vi "NTViewerUI.vi"(9 "Client Name":string, 10 "Server IP Address":string="localhost", 11 "StopNotifier":refnum<notifier>) -> ()   [LabVIEW 2015]
panel:
  in  "Tab Control":enum32{"All Table Entries", "User Page 1"}(tab)
  in  "NT Entries":string(tree)
  in  "Robot223/MyDouble2":dbl
  out "MyDouble":dbl
  # "First page of user controls. Here you can add as many controls as you like, as well as create other pages\nfor controls. These will all automatically be bound to the SmartDashboard."
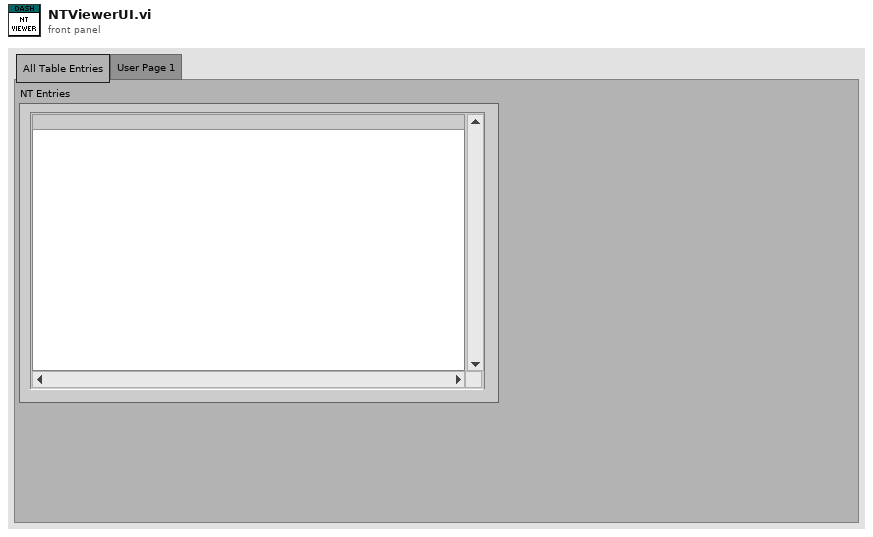
[diagram p1: front panel]
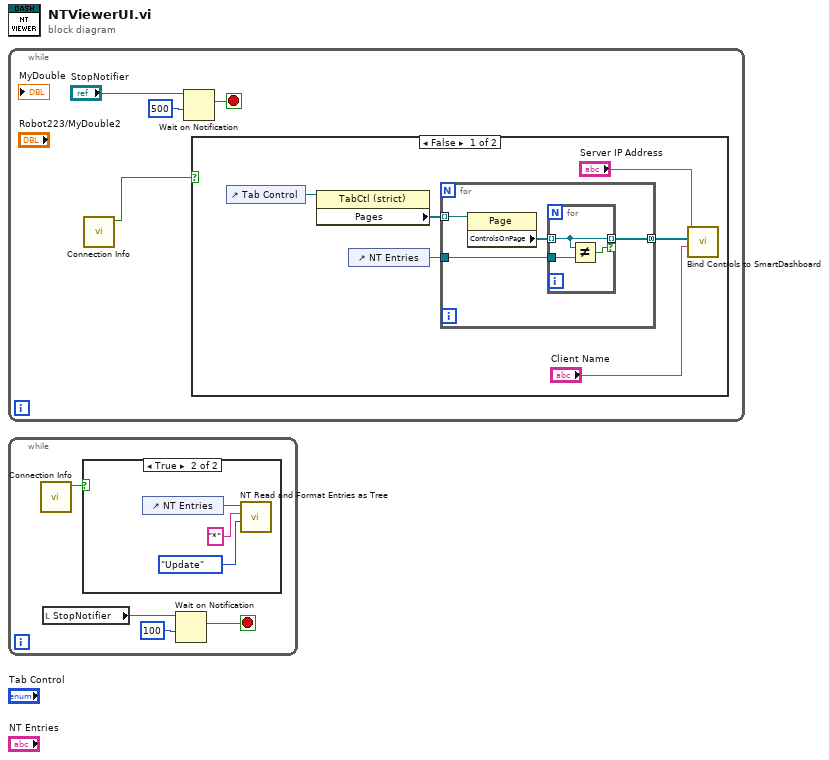
[diagram p0: block diagram]
diagram:
  n1 = while {
    stop <- w2 stop-if-true
    n2 = call <vilib>:"Connection Info.vi"() -> ("Connected"=w1:bool)  [unwired: 10 in, 1 out]
    n3 = Wait on Notification(notifier="StopNotifier", timeout in ms (-1)=500) -> (notification=w2:bool)  [unwired: 2 in, 3 out]
    n4 = case shown="False" w1 {
      frame False {
        n5 = control-ref of="Tab Control"() -> (w10:refnum<vi>)
        n6 = property class="TabCtl (strict)"(reference=w10) -> ("Pages"=w9:refnum<vi>[])  [unwired: 1 in, 2 out]
        n7 = control-ref of="NT Entries"() -> (w8:refnum<vi>)
        n8 = for {
          tunnel: w9 -> [w14] mode=indexing
          tunnel: w8 -> [w13]
          tunnel: [w11] -> w7 mode=concatenating
          n9 = property class="Page"(reference=w14) -> ("ControlsOnPage"=w12:refnum<vi>[])  [unwired: 1 in, 2 out]
          n10 = for {
            tunnel: w12 -> [w16] mode=indexing
            tunnel: w13 -> [w17]
            tunnel: [w16] -> w11 mode=indexing if=w15
            n11 = Not Equal?(x=w16, y=w17) -> (x != y?=w15:bool)
          }
        }
        n12 = call <vilib>:"Bind Controls to SmartDashboard.vi"("Path Prefix"="Client Name", "Bound Control Refs"=w7, "Server IP Address"="Server IP Address") -> ()  [unwired: 9 in]
      }
      frame True {
      }
    }
  }
  n13 = while {
    stop <- w19 stop-if-true
    n14 = call <vilib>:"Connection Info.vi"() -> ("Connected"=w18:bool)  [unwired: 10 in, 1 out]
    n15 = local read "StopNotifier"() -> (w20:refnum<notifier>)
    n16 = case shown="True" w18 {
      frame False {
      }
      frame True {
        n17 = control-ref of="NT Entries"() -> (w24:refnum<vi>)
        n18 = call <vilib>:"NT Read and Format Entries as Tree.vi"("Operation"=enum16{"Update", "Clear"}."Update", "Name Pattern"="*", "Tree Refnum"=w24) -> ()  [unwired: 7 in, 2 out]
      }
    }
    n19 = Wait on Notification(notifier=w20, timeout in ms (-1)=100) -> (notification=w19:bool)  [unwired: 2 in, 3 out]
  }
